vi "Global Write Enable.vi"(8 "error in":errorcluster, 10 "Input":enum16{"NONE", "RAM", "OFF"}(ring), 11 "PPT in":refnum<class "PPT.lvclass">) -> (0 "error out":errorcluster, 3 "PPT out":refnum<class "PPT.lvclass">)   [LabVIEW 2014, in "PPT Library.lvlib" / "PPT.lvclass"]
uses:
  PPT.lvclass
  reusable/Session APIs/Serial/Serial Session.lvclass
  PPT.lvclass/PPT.ctl
  reusable/Session APIs/Serial/Public/Asynchronous Write.vi
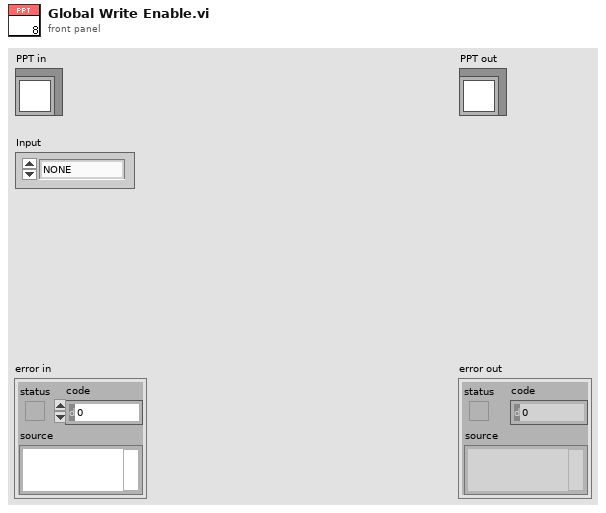
[diagram p1: front panel]
types:
  T1 = typedef "Session - Root.lvclass/Session Handle.ctl" = refnum<data-value>
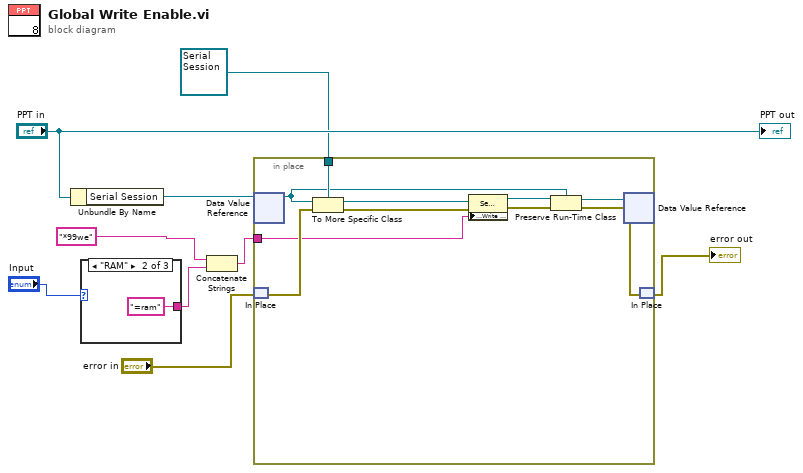
[diagram p0: block diagram]
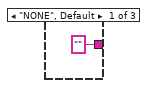
[diagram p2: hidden frame]
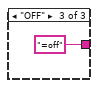
[diagram p3: hidden frame]
diagram:
  n1 = Unbundle By Name("PPT in") -> ("Serial Session"=w8:T1)
  n2 = case shown="\"RAM\"" "Input" {
    tunnel: ["" "=ram" "=off"] -> w3
    frame "NONE", Default {
    }
    frame "RAM" {
    }
    frame "OFF" {
    }
  }
  n3 = Concatenate Strings("*99we", w3) -> (w1:string)
  n4 = in-place {
    in-place-border: refnum<class "Serial Session.lvclass"> refnum ("Serial Session") -> [w21]
    in-place-border: w1 -> [w13]
    n5 = in-place-dvr #1(w8) -> (w17:refnum<class "Session - Root.lvclass">)  [unwired: 1 out]
    n6 = in-place-match #2("error in") -> (w19:errorcluster)
    n7 = To More Specific Class(target class=w21, reference=w17, error in=w19) -> (specific class reference=w20:refnum<class "Serial Session.lvclass">, error out=w22:errorcluster)
    n8 = property class="Serial Session"(reference=w20, error in=w22, "Public:Write - Asynchronous"=w13) -> (reference out=w18:refnum<class "Serial Session.lvclass">, error out=w15:errorcluster)
    n9 = Preserve Run-Time Class(object in=w18, error in=w15, 2:w17) -> (object out=w16:refnum<class "Session - Root.lvclass">, error out=w14:errorcluster)
    n10 = in-place-dvr #1(w16) -> ()  [unwired: 2 out]
    n11 = in-place-match #2(w14) -> (→"error out":errorcluster)
  }
  "PPT out" <- "PPT in"
